vi "set operation mode.vi"(8 "error in (no error)":errorcluster, 11 "CCDCamera in":refnum<class "Simulated Camera.lvclass">) -> (0 "error out":errorcluster, 3 "CCDCamera out":refnum<class "Simulated Camera.lvclass">)   [LabVIEW 2018, in "Simulated Camera.lvclass"]
uses:
  Simulated Camera.lvclass
  Simulated Camera.lvclass/Simulated Camera.ctl
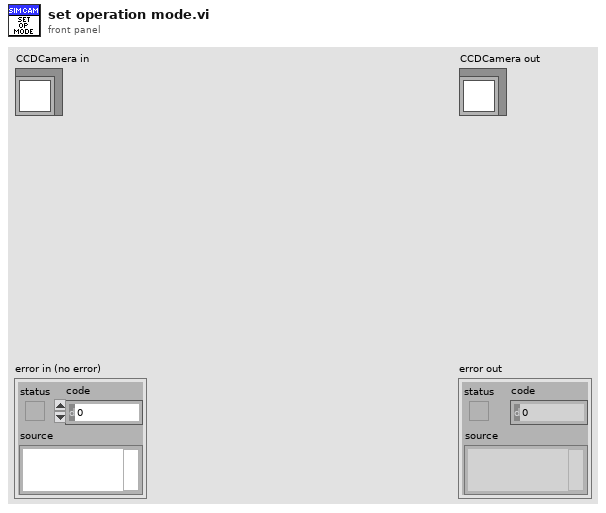
[diagram p1: front panel]
types:
  T1 = cluster{"PREAMP":u16, "READOUT_RATE":u16, "VERTICAL_SHIFT_SPEED":u16, "READ_MODE":u16, "VERTICAL_CLOCK_VOLTAGE":u16, "ACQUISITION_MODE":u16, "AD_CHANNEL":u16, "SHUTTER_TTL":u16, "SHUTTER_OPENING_TIME":u16, "SHUTTER_CLOSING_TIME":u16, "SHUTTER_MODE":u16, "TRIGGER_MODE":u16, "VBIN":u16, "INITIAL_LINE":u16, "INITIAL_COLUMN":u16, "FINAL_LINE":u16, "FINAL_COLUMN":u16, "HBIN":u16, "TEMP":u16, "COOLER_POWER_STATUS":u16}
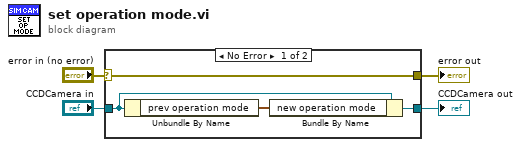
[diagram p0: block diagram]
diagram:
  n1 = case shown="No Error" "error in (no error)" {
    selector: "error in (no error)" -> [w8 w10]
    tunnel: [w8 w10] -> w4
    tunnel: [w6 w9] -> w1
    tunnel: "CCDCamera in" -> [w7 w9]
    frame No Error {
      n2 = Unbundle By Name(w7) -> ("prev operation mode"=w5:T1)
      n3 = Bundle By Name(cluster=w7, "new operation mode"=w5) -> (w6:refnum<class "Simulated Camera.lvclass">)
    }
    frame Error {
    }
  }
  "error out" <- w4
  "CCDCamera out" <- w1
